vi "Measurement UI.vi"() -> ()   [LabVIEW 2021, in "Single Tone Power Sweep_UI.lvlib"]
uses:
  Single Tone Power Sweep_UI.lvlib
  shared/controls/units - snr.ctl
  shared/controls/units - ratio.ctl
  shared/controls/digital output level units.ctl
  shared/ui/controls/view.ctl
  shared/controls/power measurement method.ctl
  UI State.ctl
  <vilib>/Utility/miscctls.llb/LVBoundsTypeDef.ctl
  <vilib>/Utility/miscctls.llb/LVPoint32TypeDef.ctl
  <vilib>/Utility/miscctls.llb/LVPointTypeDef.ctl
  shared/ui/UI Helpers.lvlib
  shared/audio popup ui/Audio Popup UI.lvlib
  shared/controls/audio controls.lvlib
panel:
  in  "xy graph meas":enum32{"THD+N", "THD", "SNR"}(ring) caption="xy"
  in  "view legend":T1
  out "plot point":string
  out "Sweep graph":cluster{"frequency (Hz)":dbl[], "THD+N":dbl[]}[](graph)
  out "Time domain graph":waveform(dbl)[](graph)
  out "Frequency domain graph":cluster{"f0":dbl, "df":dbl, "data":dbl[]}[](graph)
  out "THD":dbl[](array[numeric])
  out "THD+N":dbl[](array[numeric])
  out "SNR":dbl[](array[numeric])
  out "channel names":string[](array[string])
  in  "digital serial cfg file":string
  in  "power measurement resource":string="PXI1Slot4/ai0"
  out "efficiency (%)":dbl[](array[numeric])
  out "power loss (W)":dbl[](array[numeric])
  out "total output power (W)":dbl[](array[numeric])
  out "input power (W)":dbl[](array[numeric])
  out "power supply current (A)":dbl[](array[numeric])
  out "power supply voltage (V)":dbl[](array[numeric])
  in  "Configuration tab":enum32{"Protocol", "Measurement", "Units"}(tab)
  out "digital serial file name":string
  in  "configure digital serial":bool
  in  "master clock channel list":string caption="Master Clock Channel"
  in  "digital channel list":string caption="Digital Audio Channel"
  in  "output level units 2":T2
  in  "sense resistor (Ohms)":dbl caption="Sense Resistor" format="%#_g Ohms"
  in  "power supply current limit":dbl caption="Current Limit" format="%#_g A"
  in  "power supply voltage":dbl caption="Power Supply Voltage" format="%#_g V"
  in  "power meas resource":refnum<k15> caption="Resource"
  in  "power measurement method":T3 caption="Method"
  in  "output level units":T2
  in  "min settling cycles":u32 caption="Minimum settling cycles"
  in  "min settling time (s)":dbl=0.1 caption="Minimum settling time" format="%#_6ps"
  in  "output sweep number of steps":u32=20000 caption="Number of steps"
  in  "output level start":dbl=20.0 caption="Sweep start" format="%#_6p"
  in  "output level stop":dbl=20000.0 caption="Sweep stop"
  in  "min measurement cycles":u32 caption="Minimum measurement cycles"
  in  "Acquisition channel":tag
  in  "acq sampling rate":dbl=51200.0 caption="Sample rate" format="%#.6pHz"
  in  "min measurement time (s)":dbl=0.1 caption="Minimum measurement time" format="%#_6ps"
  in  "lowpass filter":T4(ring) caption="Lowpass filter"
  in  "highpass filter":enum32{"DC", "AC"}(ring) caption="Highpass filter"
  in  "band start":dbl=20.0 caption="Band start" format="%#_6pHz"
  in  "band stop":dbl=20000.0 caption="Band stop" format="%#_6pHz"
  in  "weighting filter":T5(ring)=enum."A-weighting" caption="Weighting filter"
  in  "load impedance":dbl=4.0 caption="Load impedance" format="%#_6p Ohms"
  in  "output range (pk-pk)":dbl=15.0 caption="Output range" format="%.3p Vpk-pk"
  in  "THD units":T6 caption="THD"
  in  "THD+N units":T6 caption="THD+N"
  in  "SNR units":T7 caption="SNR"
  in  "channel 0 offset":u32=1
  out "fft - data":dbl[](array[numeric])
  out "fft - df":dbl
  out "fft - f0":dbl
  out "wfm - data":dbl[](array[numeric])
  out "wfm - dt":dbl
  out "wfm - t0":dbl
  in  "acq channel":string="PXI1Slot4/ai0"
  in  "signal phase":dbl caption="phase"
  # "hidden controls - used to sync with MeasLink"
  # "hidden indicators"
  # "Digital Serial Settings"
  # "Harware Resource"
  # "Output Sweep"
  # "Filters"
  # "Acquisition"
  # "Power"
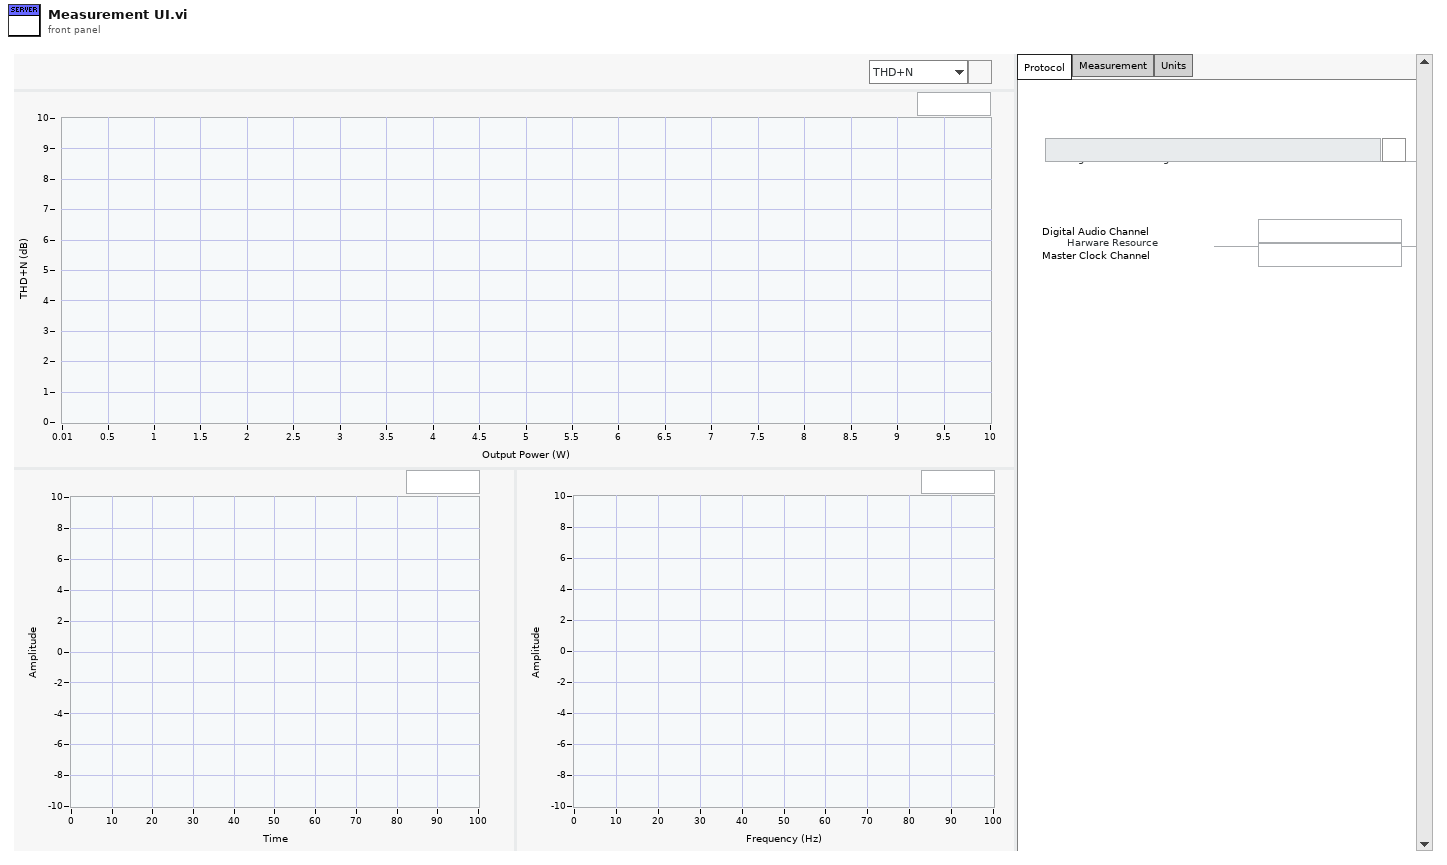
[diagram p1: front panel]
types:
  T1 = typedef "UI Helpers.lvlib/view.ctl" = bool
  T2 = typedef "audio controls.lvlib/digital output level units.ctl" = enum32{"% FS", "dBFS", "V"}
  T3 = typedef "power measurement method.ctl" = enum32{"SMU", "DMM"}
  T4 = enum32{"No filter", "AES17 20kHz", "AES17 40kHz"}
  T5 = enum32{"Linear", "A-weighting", "B-weighting", "C-weighting"}
  T6 = typedef "audio controls.lvlib/units - ratio.ctl" = enum32{"dB", "%", "x/y"}
  T7 = typedef "audio controls.lvlib/units - snr.ctl" = enum32{"dB", "x/y"}
  T8 = typedef "Single Tone Power Sweep_UI.lvlib/UI State.ctl" = cluster{"Graph Size":T9, "Legend Visible":bool, "Mouse Coords":T10, "Visible Plot Id":i32, "PostUI event occurred":bool, "digital serial cfg file":path}
  T9 = typedef "LVBoundsTypeDef.ctl" = cluster{"Width":u32, "Height":u32}
  T10 = typedef "LVPoint32TypeDef.ctl" = cluster{"Horizontal":i32, "Vertical":i32}
  T11 = typedef "LVPointTypeDef.ctl" = cluster{"Horizontal":i16, "Vertical":i16}
  T12 = typedef "Audio Popup UI.lvlib/audio settings.ctl" = cluster{"digital serial file":string}
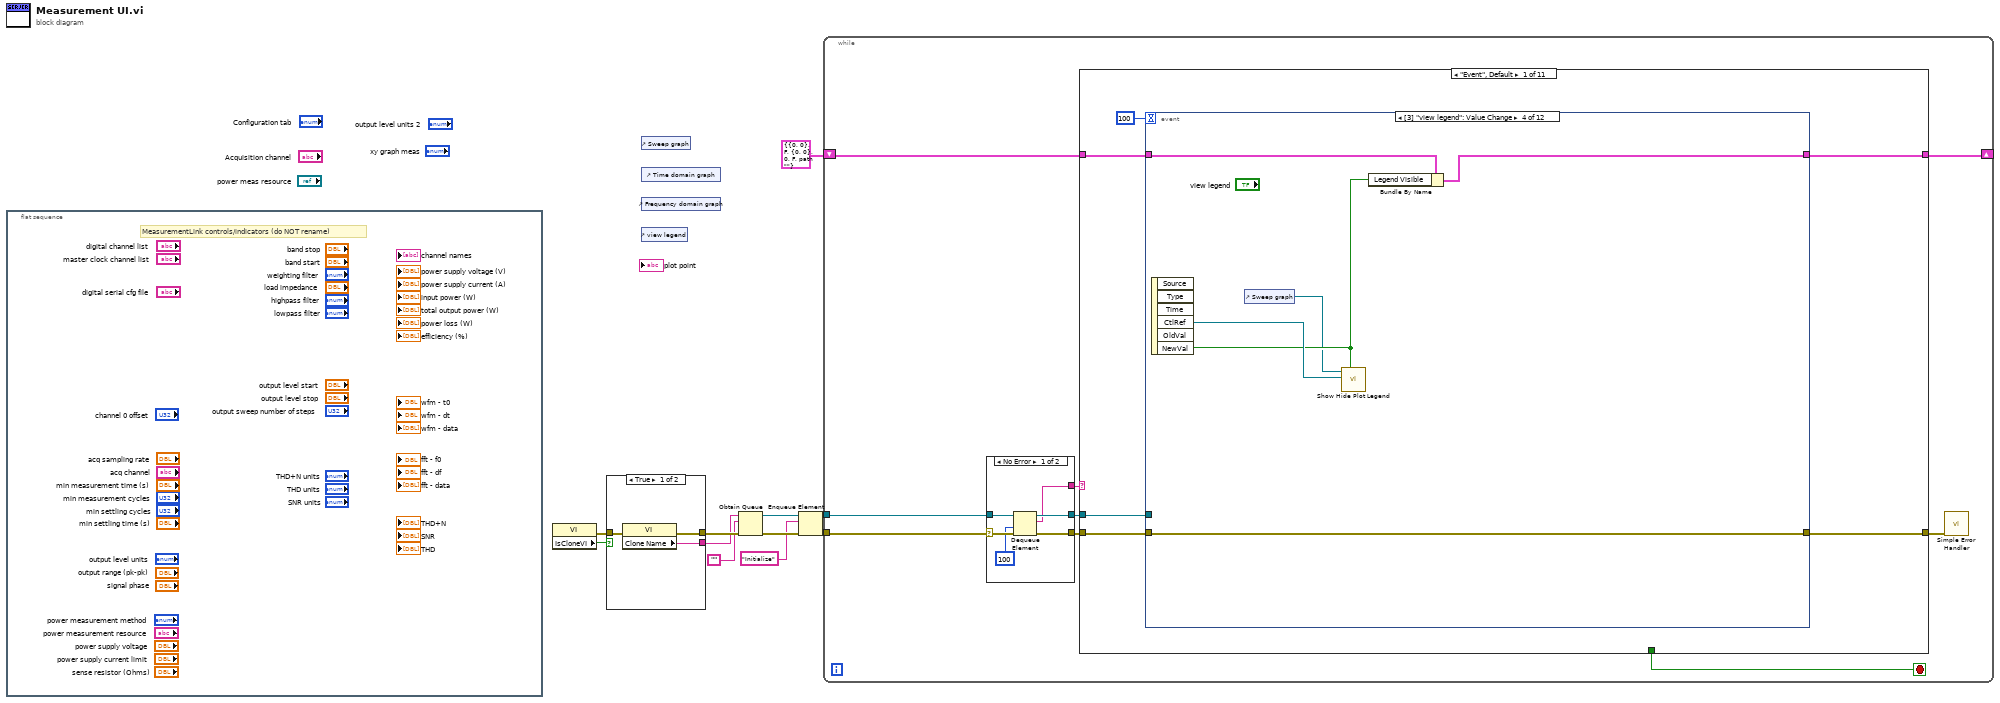
[diagram p0: block diagram]
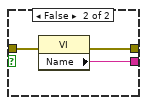
[diagram p2: hidden frame]
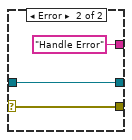
[diagram p3: hidden frame]
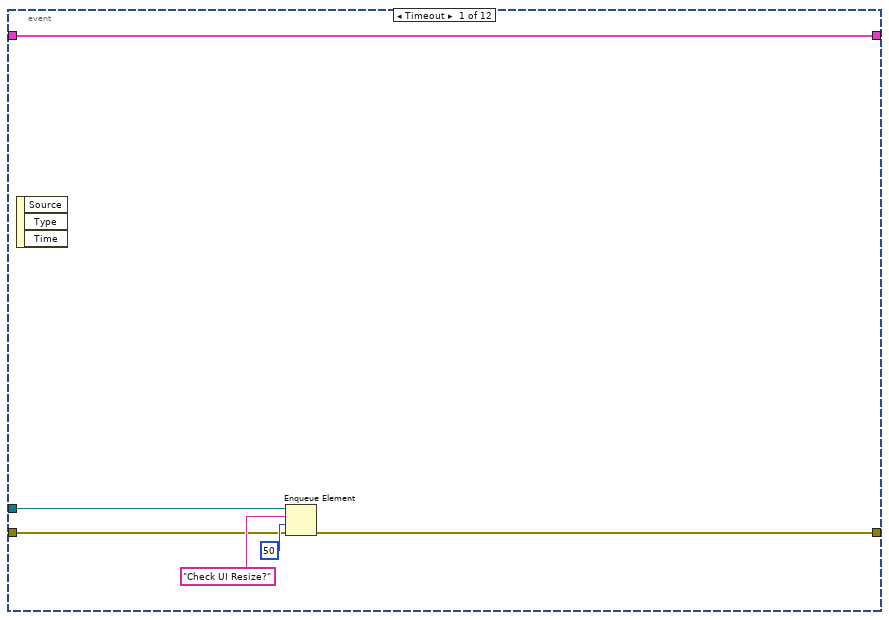
[diagram p4: hidden frame]
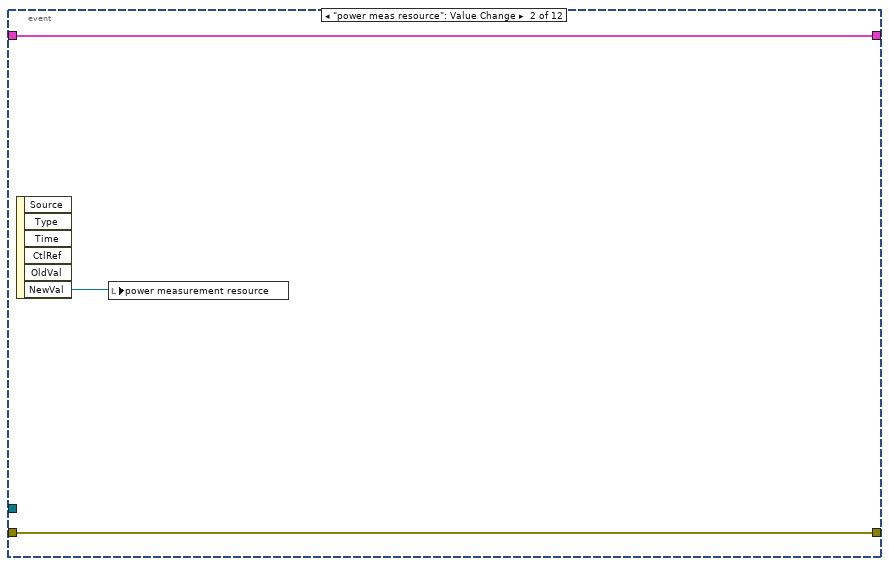
[diagram p5: hidden frame]
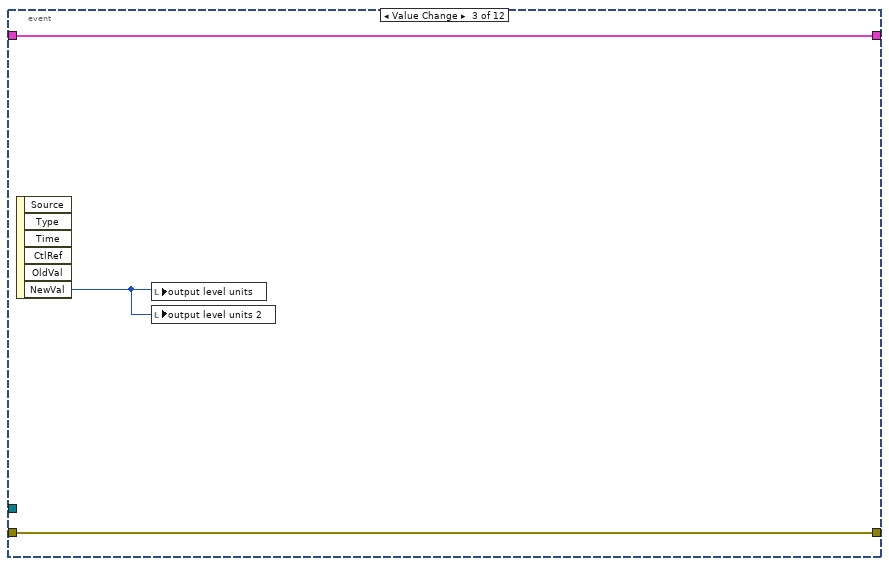
[diagram p6: hidden frame]
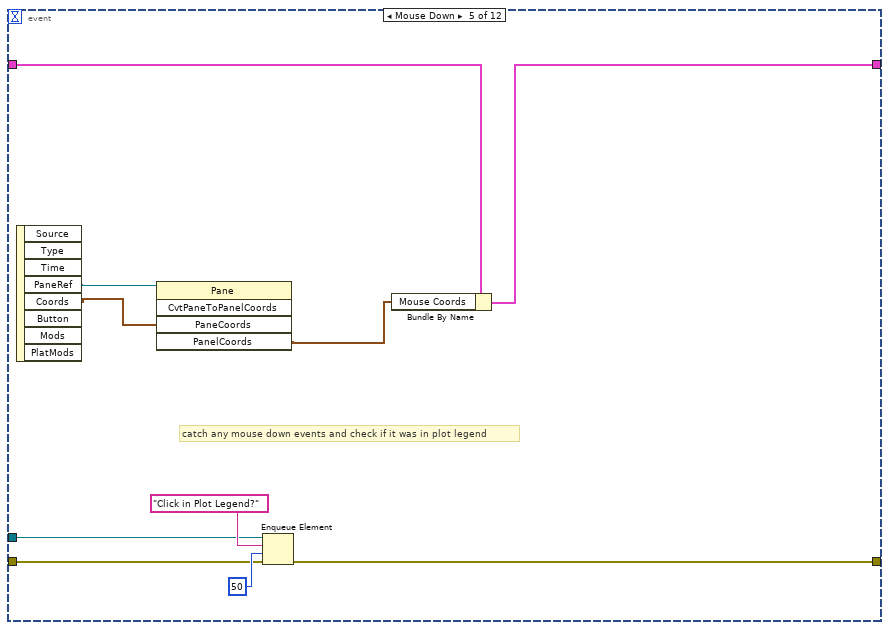
[diagram p7: hidden frame]
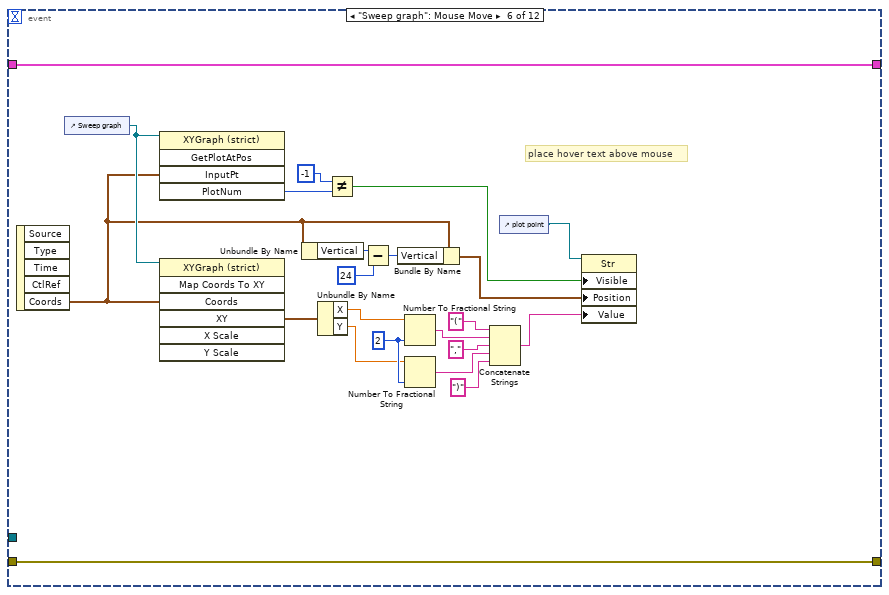
[diagram p8: hidden frame]
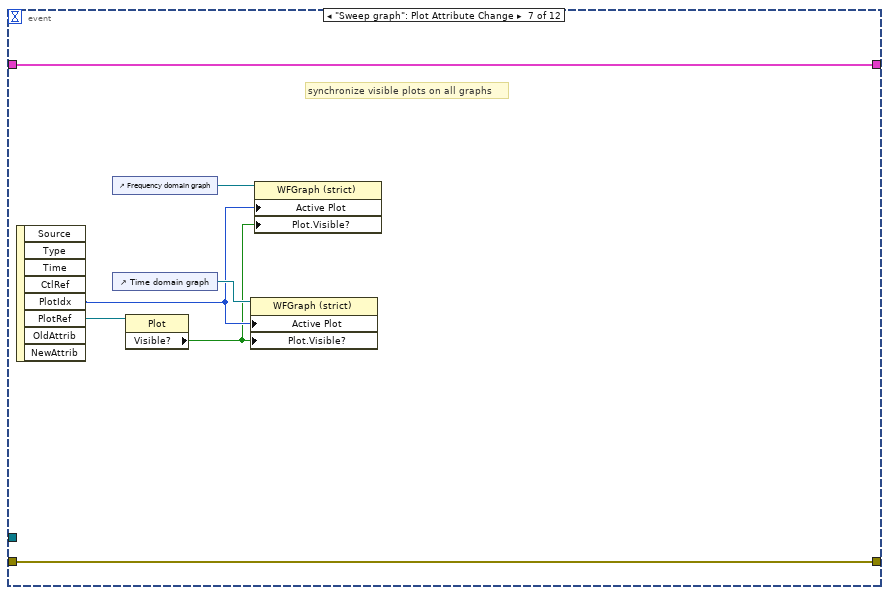
[diagram p9: hidden frame]
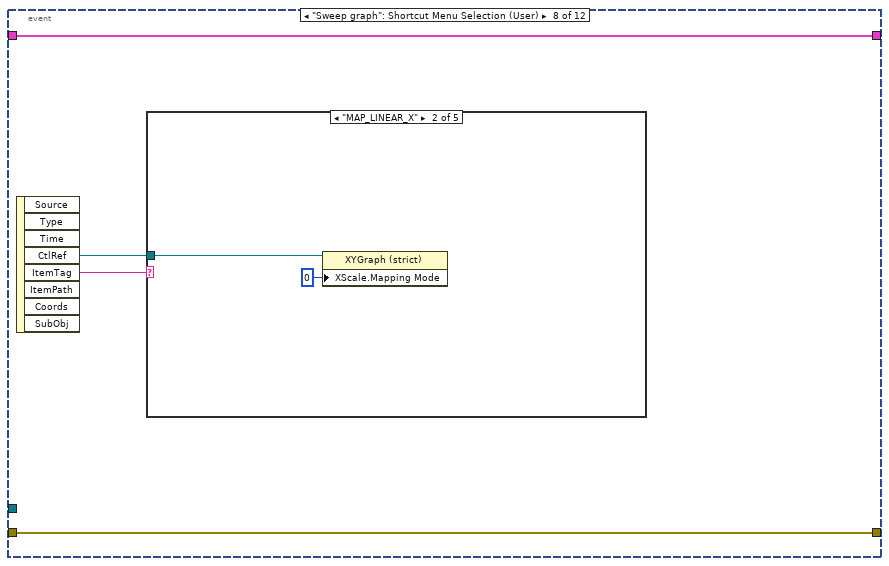
[diagram p10: hidden frame]
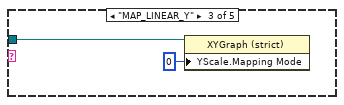
[diagram p12: hidden frame]
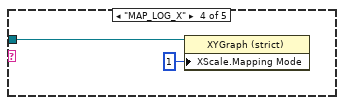
[diagram p13: hidden frame]
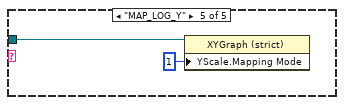
[diagram p14: hidden frame]
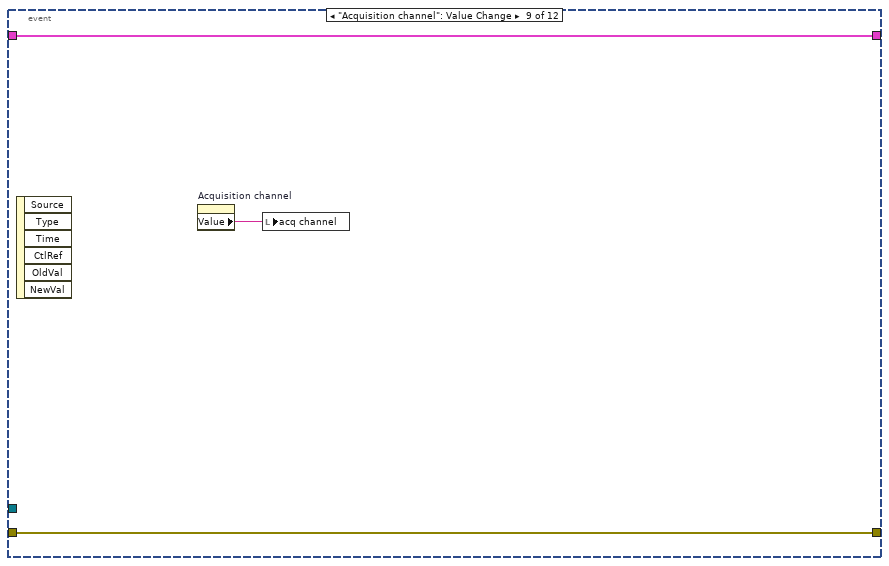
[diagram p15: hidden frame]
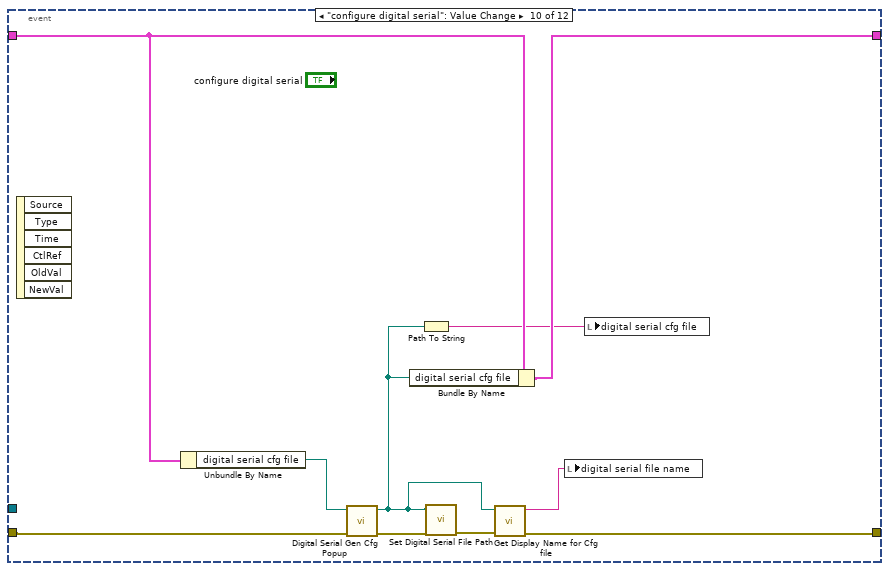
[diagram p16: hidden frame]
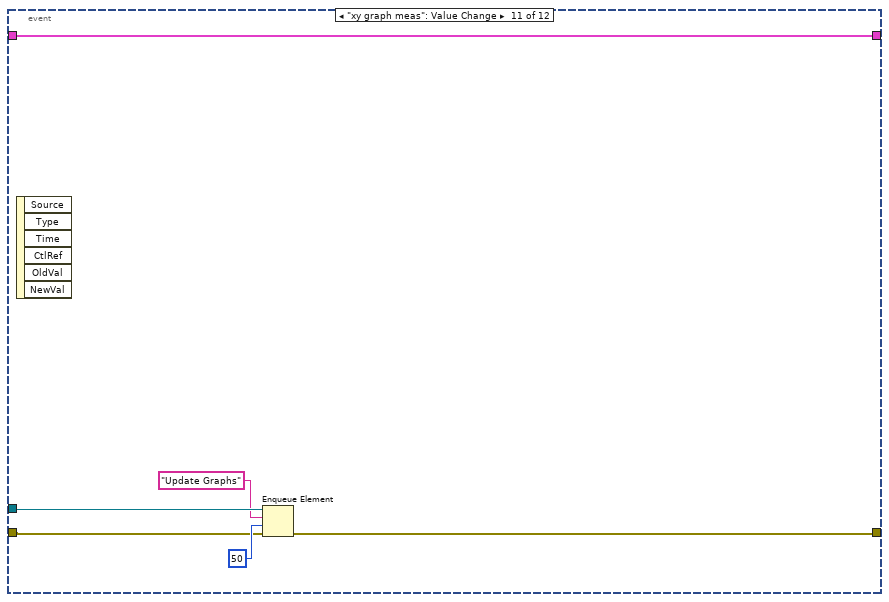
[diagram p17: hidden frame]
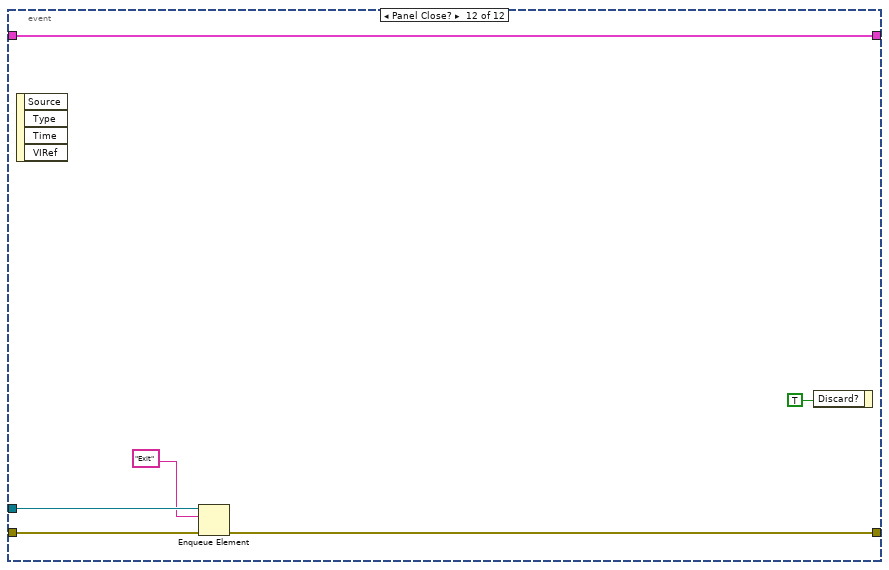
[diagram p18: hidden frame]
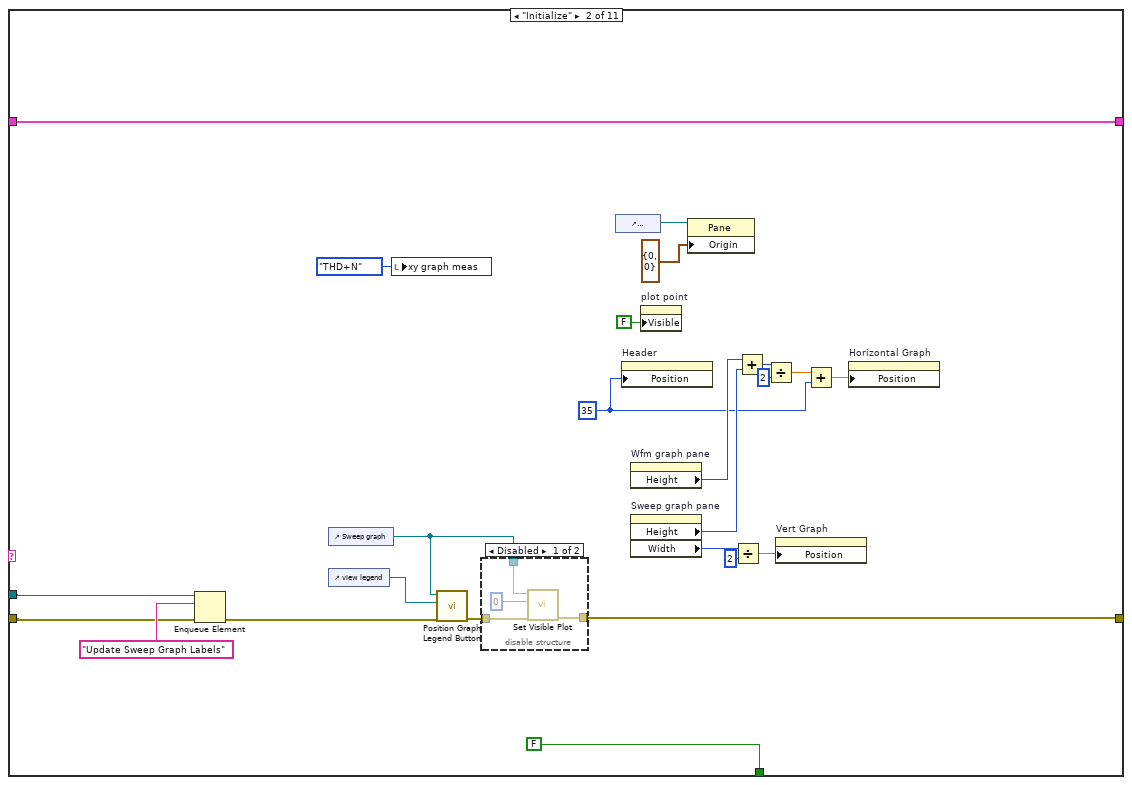
[diagram p19: hidden frame]
diagram:
  n1 = flat-sequence {
    frame #0 {
      # "MeasurementLink controls/indicators (do NOT rename)"
    }
  }
  n2 = property class="VI"() -> (error out=w2:errorcluster, "IsCloneVI"=w3:bool)  [unwired: 2 in, 1 out]
  n3 = case shown="True" w3 {
    tunnel: [w14 w17] -> w11
    tunnel: [w13 w16] -> w10
    tunnel: w2 -> [w12 w15]
    frame True {
      n4 = property class="VI"(error in=w12) -> (error out=w14:errorcluster, "Clone Name"=w13:string)  [unwired: 1 in, 1 out]
    }
    frame False {
      n5 = property class="VI"(error in=w15) -> (error out=w17:errorcluster, "Name"=w16:string)  [unwired: 1 in, 1 out]
    }
  }
  n6 = control-ref of="Sweep graph"() -> ()  [unwired: 1 out]
  n7 = control-ref of="Time domain graph"() -> ()  [unwired: 1 out]
  n8 = control-ref of="Frequency domain graph"() -> ()  [unwired: 1 out]
  n9 = control-ref of="view legend"() -> ()  [unwired: 1 out]
  n10 = Obtain Queue(name (unnamed)=w10, element data type="", error in (no error)=w11) -> (queue out=w7:refnum<queue>, error out=w9:errorcluster)  [unwired: 2 in, 1 out]
  n11 = Enqueue Element(queue=w7, element="Initialize", error in (no error)=w9) -> (queue out=w6:refnum<queue>, error out=w8:errorcluster)  [unwired: 1 in, 1 out]
  n12 = while {
    tunnel: w6 -> [w24]
    shift-right: [w20] -> _
    shift-left: T8 {"Graph Size"={"Width"=0, "Height"=0}, "Legend Visible"=FALSE, "Mouse Coords"={"Horizontal"=0, "Vertical"=0}, "Visible Plot Id"=0, "PostUI event occurred"=FALSE, "digital serial cfg file"=path ""} ("UI State") -> [w19]
    tunnel: w8 -> [w26]
    stop <- w21 stop-if-true
    n13 = case shown="No Error" w26 {
      selector: w26 -> [w32 w35]
      tunnel: [w31 w35] -> w25
      tunnel: w24 -> [w30 w34]
      tunnel: [w29 w34] -> w23
      tunnel: [w28 "Handle Error"] -> w22
      frame No Error {
        n14 = Dequeue Element(queue=w30, timeout in ms (-1)=100, error in (no error)=w32) -> (queue out=w29:refnum<queue>, element=w28:string, error out=w31:errorcluster)  [unwired: 1 out]
      }
      frame Error {
      }
    }
    n15 = case shown="\"Event\", Default" w22 {
      tunnel: w25 -> [w40 w143 w169 w193 w213 w229 w237 w266 w296 w319 w321]
      tunnel: w23 -> [w38 w144 w170 w194 _ _ w236 w267 _ w317 _]
      tunnel: [w41 w147 w168 w192 w212 w220 w231 w265 w296 w314 w321] -> w18
      tunnel: [_ FALSE _ _ _ _ _ _ _ TRUE _] -> w21
      tunnel: [w36 w137 w165 w191 w215 w230 w234 w284 w295 w312 w320] -> w20
      tunnel: w19 -> [w37 w137 w166 w191 w216 w230 w235 w284 w295 w312 w320]
      frame "Event", Default {
        n16 = event shown="[3] \"view legend\": Value Change" {
          selector: _ -> [_ _ _ _ _ _ _ _ _ _ _ _]
          dyn-events: _ -> [_ _ _ _ _ _ _ _ _ _ _ _]
          timeout: 100 -> [_ _ _ _ _ _ _ _ _ _ _ _]
          tunnel: [w44 w50 w53 w59 w65 w91 w97 w102 w111 w114 w124 w133] -> w41
          tunnel: w40 -> [w45 w50 w53 w59 w67 w91 w97 w102 w111 w119 w127 w134]
          tunnel: w38 -> [w43 _ _ _ w66 _ _ _ _ _ w126 w132]
          tunnel: w37 -> [w42 w49 w52 w56 w64 w90 w96 w101 w112 w118 w129 w130]
          tunnel: [w42 w49 w52 w55 w63 w90 w96 w101 w112 w117 w129 w130] -> w36
          event Timeout {
            n17 = event-data() -> ()  [unwired: 1 in, 3 out]
            n18 = Enqueue Element(queue=w43, element="Check UI Resize?", timeout in ms (-1)=50, error in (no error)=w45) -> (error out=w44:errorcluster)  [unwired: 2 out]
          }
          event "power meas resource": Value Change {
            n19 = event-data() -> ("NewVal"=w48:refnum<k15>)  [unwired: 1 in, 5 out]
            n20 = local write "power measurement resource"(w48) -> ()
          }
          event Value Change {
            n21 = event-data() -> ("NewVal"=w51:T2)  [unwired: 1 in, 5 out]
            n22 = local write "output level units"(w51) -> ()
            n23 = local write "output level units 2"(w51) -> ()
          }
          event Value Change {
            n24 = event-data() -> ("CtlRef"=w58:refnum<vi>, "NewVal"=w57:T1)  [unwired: 1 in, 4 out]
            n25 = control-ref of="Sweep graph"() -> (w54:refnum<vi>)
            n26 = call "Show Hide Plot Legend.vi"("show"=w57, "view reference"=w58, "graph reference"=w54) -> ()  [unwired: 8 in, 1 out]
            n27 = Bundle By Name(cluster=w56, "Legend Visible"=w57) -> (w55:T8)
          }
          event Mouse Down {
            # "catch any mouse down events and check if it was in plot legend"
            n28 = event-data() -> ("PaneRef"=w62:refnum<vi>, "Coords"=w61:T10)  [unwired: 1 in, 6 out]
            n29 = invoke class="Pane" method="CvtPaneToPanelCoords"(reference=w62, "PaneCoords"=w61) -> ("PanelCoords"=w60:T11)  [unwired: 3 in, 4 out]
            n30 = Enqueue Element(queue=w66, element="Click in Plot Legend?", timeout in ms (-1)=50, error in (no error)=w67) -> (error out=w65:errorcluster)  [unwired: 2 out]
            n31 = Bundle By Name(cluster=w64, "Mouse Coords"=w60) -> (w63:T8)
          }
          event "Sweep graph": Mouse Move {
            w80 = i16 2 ("precision (6)")
            # "place hover text above mouse"
            n32 = event-data() -> ("Coords"=w70:T10)  [unwired: 1 in, 4 out]
            n33 = control-ref of="Sweep graph"() -> (w71:refnum<vi>)
            n34 = invoke class="XYGraph (strict)" method="GetPlotAtPos"(reference=w71, "InputPt"=w70) -> ("PlotNum"=w88:i32)  [unwired: 3 in, 4 out]
            n35 = invoke class="XYGraph (strict)" method="Map Coords To XY"(reference=w71, "Coords"=w70) -> ("XY"=w89:cluster{"X":dbl, "Y":dbl})  [unwired: 5 in, 6 out]
            n36 = Unbundle By Name(w70) -> ("Vertical"=w75:i32)
            n37 = Unbundle By Name(w89) -> ("X"=w78:dbl, "Y"=w77:dbl)
            n38 = Not Equal?(x=-1, y=w88) -> (x != y?=w86:bool)
            n39 = Subtract(x=w75, y=24) -> (x-y=w74:i32)
            n40 = Bundle By Name(cluster=w70, "Vertical"=w74) -> (w76:T10)
            n41 = Number To Fractional String(number=w78, precision (6)=w80) -> (F-format string=w84:string)  [unwired: 2 in]
            n42 = Number To Fractional String(number=w77, precision (6)=w80) -> (F-format string=w82:string)  [unwired: 2 in]
            n43 = Concatenate Strings("(" ("string"), w84, "," ("string"), w82, ")" ("string")) -> (w79:string)
            n44 = control-ref of="plot point"() -> (w72:refnum<vi>)
            n45 = property on="Property Node" class="Str"(reference=w72, "Visible"=w86, "Position"=w76, "Value"=w79) -> ()  [unwired: 1 in, 2 out]
          }
          event "Sweep graph": Plot Attribute Change {
            # "synchronize visible plots on all graphs"
            n46 = event-data() -> ("PlotIdx"=w93:i32, "PlotRef"=w98:refnum<vi>)  [unwired: 1 in, 6 out]
            n47 = control-ref of="Frequency domain graph"() -> (w94:refnum<vi>)
            n48 = control-ref of="Time domain graph"() -> (w95:refnum<vi>)
            n49 = property class="Plot"(reference=w98) -> ("Visible?"=w92:bool)  [unwired: 1 in, 2 out]
            n50 = property on="Property Node" class="WFGraph (strict)"(reference=w95, "Active Plot"=w93, "Plot.Visible?"=w92) -> ()  [unwired: 1 in, 2 out]
            n51 = property on="Property Node" class="WFGraph (strict)"(reference=w94, "Active Plot"=w93, "Plot.Visible?"=w92) -> ()  [unwired: 1 in, 2 out]
          }
          event "Sweep graph": Shortcut Menu Selection (User) {
            n52 = event-data() -> ("CtlRef"=w99:refnum<vi>, "ItemTag"=w100:string)  [unwired: 1 in, 6 out]
            n53 = case shown="\"MAP_LINEAR_X\"" w100 {
              tunnel: w99 -> [_ w104 w106 w108 w110]
              frame "", Default {
              }
              frame "MAP_LINEAR_X" {
                n54 = property class="XYGraph (strict)"(reference=w104, "XScale.Mapping Mode"=u8 0 ("X Scale.Mapping Mode")) -> ()  [unwired: 1 in, 2 out]
              }
              frame "MAP_LINEAR_Y" {
                n55 = property class="XYGraph (strict)"(reference=w106, "YScale.Mapping Mode"=u8 0 ("X Scale.Mapping Mode")) -> ()  [unwired: 1 in, 2 out]
              }
              frame "MAP_LOG_X" {
                n56 = property class="XYGraph (strict)"(reference=w108, "XScale.Mapping Mode"=u8 1 ("X Scale.Mapping Mode")) -> ()  [unwired: 1 in, 2 out]
              }
              frame "MAP_LOG_Y" {
                n57 = property class="XYGraph (strict)"(reference=w110, "YScale.Mapping Mode"=u8 1 ("X Scale.Mapping Mode")) -> ()  [unwired: 1 in, 2 out]
              }
            }
          }
          event "Acquisition channel": Value Change {
            n58 = event-data() -> ()  [unwired: 1 in, 6 out]
            n59 = property on="Acquisition channel" class="DAQmxName"() -> ("Value"=w113:string)  [unwired: 2 in, 2 out]
            n60 = local write "acq channel"(w113) -> ()
          }
          event "configure digital serial": Value Change {
            n61 = event-data() -> ()  [unwired: 1 in, 6 out]
            n62 = Unbundle By Name(w118) -> ("digital serial cfg file"=w123:path)
            n63 = call "Digital Serial Gen Cfg Popup.vi"("error in (no error)"=w119, "config file in"=w123) -> ("error out"=w122:errorcluster, "config file out"=w120:path)  [unwired: 7 in, 1 out]
            n64 = Bundle By Name(cluster=w118, "digital serial cfg file"=w120) -> (w117:T8)
            n65 = Path To String(path=w120) -> (string=w116:string)
            n66 = call "Set Digital Serial File Path.vi"("error in (no error)"=w122, "digital serial file"=w120) -> ("error out"=w121:errorcluster)  [unwired: 9 in]
            n67 = call "Get Display Name for Cfg file.vi"("error in (no error)"=w121, "file path"=w120) -> ("error out"=w114:errorcluster, "display string"=w115:string)  [unwired: 8 in]
            n68 = local write "digital serial file name"(w115) -> ()
            n69 = local write "digital serial cfg file"(w116) -> ()
          }
          event "xy graph meas": Value Change {
            n70 = event-data() -> ()  [unwired: 1 in, 6 out]
            n71 = Enqueue Element(queue=w126, element="Update Graphs", timeout in ms (-1)=50, error in (no error)=w127) -> (error out=w124:errorcluster)  [unwired: 2 out]
          }
          event Panel Close? {
            n72 = event-data() -> ()  [unwired: 1 in, 4 out]
            n73 = Enqueue Element(queue=w132, element="Exit", error in (no error)=w134) -> (error out=w133:errorcluster)  [unwired: 1 in, 2 out]
            n74 = event-data("Discard?"=TRUE) -> ()  [unwired: 1 in, 1 out]
          }
        }
      }
      frame "Initialize" {
        w141 = 35 ("Splitter Position")
        n75 = Enqueue Element(queue=w144, element="Update Sweep Graph Labels", error in (no error)=w143) -> (error out=w142:errorcluster)  [unwired: 1 in, 2 out]
        n76 = control-ref of="Sweep graph"() -> (w146:refnum<vi>)
        n77 = control-ref of="view legend"() -> (w158:refnum<vi>)
        n78 = local write "xy graph meas"(enum32{"THD+N", "THD", "SNR"}."THD+N" ("xy graph meas")) -> ()
        n79 = call "Position Graph Legend Button.vi"("error in (no error)"=w142, "view legend"=w158, "graph"=w146) -> ("error out"=w148:errorcluster)  [unwired: 8 in]
        n80 = disable-structure shown="Disabled" {
          disable-tunnel: w148 -> [w163 w164]
          disable-tunnel: [w162 w164] -> w147
          disable-tunnel: w146 -> [w161 _]
          frame Disabled {
            n81 = call "Set Visible Plot.vi"("error in (no error)"=w163, "Plot Id"=0, "XYGraph in"=w161) -> ("error out"=w162:errorcluster)  [unwired: 8 in]
          }
          frame Enabled {
          }
        }
        n82 = control-ref of="Configuration Pane"() -> (w140:refnum<vi>)
        n83 = property on="Header" class="Splitter"("Position"=w141) -> ()  [unwired: 2 in, 2 out]
        n84 = property on="Wfm graph pane" class="Pane"() -> ("Height"=w151:u32)  [unwired: 2 in, 2 out]
        n85 = property on="Sweep graph pane" class="Pane"() -> ("Height"=w150:u32, "Width"=w153:u32)  [unwired: 2 in, 2 out]
        n86 = property on="plot point" class="Str"("Visible"=FALSE) -> ()  [unwired: 2 in, 2 out]
        n87 = property class="Pane"(reference=w140, "Origin"=T11 {"Horizontal"=0, "Vertical"=0}) -> ()  [unwired: 1 in, 2 out]
        n88 = Divide(x=w153, y=2) -> (x/y=w152:dbl)
        n89 = Add(x=w151, y=w150) -> (x+y=w149:u32)
        n90 = Divide(x=w149, y=2) -> (x/y=w156:dbl)
        n91 = property on="Vert Graph" class="Splitter"("Position"=w152) -> ()  [unwired: 2 in, 2 out]
        n92 = Add(x=w156, y=w141) -> (x+y=w155:dbl)
        n93 = property on="Horizontal Graph" class="Splitter"("Position"=w155) -> ()  [unwired: 2 in, 2 out]
      }
      frame "Check UI Resize?" {
        n94 = control-ref of="Time domain graph"() -> (w167:refnum<vi>)
        n95 = property on="Property Node" class="WFGraph (strict)"(reference=w167, error in=w169) -> (error out=w175:errorcluster, "Bounds"=w171:T9)  [unwired: 1 out]
        n96 = Unbundle By Name(w166) -> ("Legend Visible"=w173:bool, "Graph Size"=w172:T9)
        n97 = Not Equal?(x=w172, y=w171) -> (x != y?=w174:bool)
        n98 = Bundle By Name(cluster=w166, "Graph Size"=w171) -> (w165:T8)
        n99 = case shown="True" w174 {
          tunnel: w175 -> [w176 w183]
          tunnel: [w176 w178] -> w168
          tunnel: w173 -> [_ w181]
          tunnel: w170 -> [_ w182]
          frame False {
            # "no resize"
          }
          frame True {
            # "panel resized"
            n100 = case shown="True" w181 {
              tunnel: w183 -> [w185 w190]
              tunnel: [w185 w189] -> w180
              tunnel: w182 -> [w184 w188]
              tunnel: [w184 w186] -> w179
              frame False {
              }
              frame True {
                n101 = Enqueue Element(queue=w188, element="Hide Plot Legend", error in (no error)=w190) -> (queue out=w186:refnum<queue>, error out=w189:errorcluster)  [unwired: 1 in, 1 out]
              }
            }
            n102 = Enqueue Element(queue=w179, element="Panel Resize", error in (no error)=w180) -> (error out=w178:errorcluster)  [unwired: 1 in, 2 out]
          }
        }
      }
      frame "Click in Plot Legend?" {
        n103 = Unbundle By Name(w191) -> ("Legend Visible"=w195:bool, "Mouse Coords"=w196:T10)
        n104 = case shown="True" w195 {
          tunnel: w196 -> [_ w203]
          tunnel: w194 -> [_ w200]
          tunnel: w193 -> [w197 w204]
          tunnel: [w197 w199] -> w192
          frame False {
            # "legend not visible; do nothing"
          }
          frame True {
            # "check if mouse down in legend"
            n105 = control-ref of="Sweep graph"() -> (w198:refnum<vi>)
            n106 = call "Check if Click in Graph Legend.vi"("error in (no error)"=w204, "Mouse Coords"=w203, "WaveformGraph"=w198) -> ("error out"=w201:errorcluster, "click in legend?"=w202:bool)  [unwired: 7 in]
            n107 = case shown="True" w202 {
              tunnel: w201 -> [w208 w209]
              tunnel: w200 -> [w207 _]
              tunnel: [w206 w209] -> w199
              frame False {
                n108 = Enqueue Element(queue=w207, element="Hide Plot Legend", error in (no error)=w208) -> (error out=w206:errorcluster)  [unwired: 1 in, 2 out]
              }
              frame True {
                # "inside legend; do nothing"
              }
            }
          }
        }
      }
      frame "Hide Plot Legend" {
        n109 = control-ref of="Sweep graph"() -> (w210:refnum<vi>)
        n110 = control-ref of="view legend"() -> (w211:refnum<vi>)
        n111 = call "Show Hide Plot Legend.vi"("show"=FALSE, "error in (no error)"=w213, "view reference"=w211, "graph reference"=w210) -> ("error out"=w212:errorcluster)  [unwired: 7 in]
        n112 = Bundle By Name(cluster=w216, "Legend Visible"=FALSE ("legend visible")) -> (w215:T8)
      }
      frame "Panel Resize" {
        # "align 'xy meas selection' with 'view legend' boolean"
        n113 = control-ref of="Sweep graph"() -> (w228:refnum<vi>)
        n114 = control-ref of="view legend"() -> (w226:refnum<vi>)
        n115 = call "Position Graph Legend Button.vi"("error in (no error)"=w229, "view legend"=w226, "graph"=w228) -> ("error out"=w227:errorcluster)  [unwired: 8 in]
        n116 = property on="Property Node" class="Bool (strict)"(reference=w226, error in=w227) -> (error out=w224:errorcluster, "Left"=w219:i32)  [unwired: 1 out]
        n117 = control-ref of="xy graph meas"() -> (w225:refnum<vi>)
        n118 = property class="Enum (strict)"(reference=w225, error in=w224) -> (reference out=w223:refnum<vi>, error out=w222:errorcluster, "Width"=w218:u32)
        n119 = Subtract(x=w219, y=w218) -> (x-y=w221:u32)
        n120 = property class="Enum (strict)"(reference=w223, error in=w222, "Left"=w221) -> (error out=w220:errorcluster)  [unwired: 1 out]
      }
      frame "Post UI Update" {
        # "This case will be triggered, after framework updates the User interface with result values."
        n121 = for {
          tunnel: w236 -> [w262]
          shift-right: [w261] -> w232
          shift-left: w237 -> [w263]
          tunnel: string[] ["Update Graphs"] -> [w260] mode=indexing
          n122 = Enqueue Element(queue=w262, element=w260, timeout in ms (-1)=50, error in (no error)=w263) -> (error out=w261:errorcluster)  [unwired: 2 out]
        }
        n123 = Unbundle By Name(w235) -> ("PostUI event occurred"=w233:bool)
        n124 = case shown="False" w233 {
          tunnel: w235 -> [w251 w259]
          tunnel: [w250 w259] -> w234
          tunnel: w232 -> [w245 w258]
          tunnel: [w240 w258] -> w231
          frame False {
            # "Initialize the DAQmx channel control"
            # "do this on first PostUI Event (happens when panel loads)"
            n125 = local read "digital serial cfg file"() -> (w242:string)
            n126 = local read "power measurement resource"() -> (w248:string)
            n127 = Empty String/Path?(string/path=w242) -> (empty?=w241:bool)
            n128 = local read "acq channel"() -> (w247:string)
            n129 = case shown="True" w241 {
              tunnel: w245 -> [w253 w257]
              tunnel: [w253 w255] -> w246
              tunnel: w242 -> [w252 _]
              tunnel: [w252 w254] -> w243
              frame False {
              }
              frame True {
                n130 = call "Get Audio Settings.vi"("error in (no error)"=w257) -> ("error out"=w255:errorcluster, "audio settings"=w256:T12)  [unwired: 9 in]
                n131 = Unbundle By Name(w256) -> ("digital serial file"=w254:string)
              }
            }
            n132 = local write "power meas resource"(w248) -> ()
            n133 = property on="Acquisition channel" class="DAQmxName"("Value"=w247) -> ()  [unwired: 2 in, 2 out]
            n134 = String To Path(string=w243) -> (path=w244:path)
            n135 = local write "digital serial cfg file"(w243) -> ()
            n136 = call "Get Display Name for Cfg file.vi"("error in (no error)"=w246, "file path"=w244) -> ("error out"=w240:errorcluster, "display string"=→"digital serial file name":string)  [unwired: 8 in]
            n137 = Bundle By Name(cluster=w251, "PostUI event occurred"=TRUE, "digital serial cfg file"=w244) -> (w250:T8)
          }
          frame True {
          }
        }
      }
      frame "Update Graphs" {
        n138 = local read "channel names"() -> (w274:string[])
        n139 = disable-structure shown="Disabled" {
          frame Disabled {
            # "maybe use for debugging ???"
            n140 = local read "power supply voltage (V)"() -> ()  [unwired: 1 out]
            n141 = local read "power supply current (A)"() -> ()  [unwired: 1 out]
          }
          frame Enabled {
          }
        }
        n142 = control-ref of="Sweep graph"() -> (w283:refnum<vi>)
        n143 = Array Size(array=w274) -> (size(s)=w282:i32)
        n144 = Enqueue Element(queue=w267, element="Update Sweep Graph Labels", error in (no error)=w266) -> (error out=w265:errorcluster)  [unwired: 1 in, 2 out]
        n145 = property class="XYGraph (strict)"(reference=w283, "LegNumRows"=w282, "LegScrollVis"=FALSE ("Legend:Scrollbar Visible")) -> ()  [unwired: 1 in, 2 out]
        n146 = for {
          tunnel: w274 -> [w291] mode=indexing
          tunnel: w283 -> [w290]
          i -> [w292]
          n147 = property on="Property Node" class="XYGraph (strict)"(reference=w290, "Active Plot"=w292, "Plot.Plot Name"=w291, "Plot.Point Style"=u8 5, "Plot.Visible?"=TRUE ("Plot.Visible")) -> ()  [unwired: 1 in, 2 out]
        }
        n148 = local read "xy graph meas"() -> (w269:enum32{"THD+N", "THD", "SNR"})
        n149 = local read "fft - data"() -> (w271:dbl[])
        n150 = local read "wfm - data"() -> (w277:dbl[])
        n151 = local read "fft - df"() -> (w273:dbl)
        n152 = local read "fft - f0"() -> (w272:dbl)
        n153 = local read "wfm - dt"() -> (w276:dbl)
        n154 = local read "total output power (W)"() -> (w279:dbl[])
        n155 = case shown="\"SNR\"" w269 {
          tunnel: [w285 w286 w287] -> w278
          frame "THD+N", Default {
            n156 = local read "THD+N"() -> (w285:dbl[])
          }
          frame "THD" {
            n157 = local read "THD"() -> (w286:dbl[])
          }
          frame "SNR" {
            n158 = local read "SNR"() -> (w287:dbl[])
          }
        }
        n159 = call "Array to Wfm (N Ch).vi"("channel names"=w274, "dt"=w276, "array"=w277) -> ("waveforms"=→"Time domain graph":waveform(dbl)[])  [unwired: 8 in]
        n160 = call "Array to Spectra (N Ch).vi"("channel names"=w274, "df"=w273, "f0"=w272, "data"=w271) -> ("spectra"=→"Frequency domain graph":cluster{"f0":dbl, "df":dbl, "data":dbl[]}[])  [unwired: 7 in]
        n161 = call "Array to XY (N Ch).vi"("channel names"=w274, "Y data"=w278, "X data"=w279) -> ("XY plots"=→"Sweep graph":cluster{"X data":dbl[], "Y data":dbl[]}[])  [unwired: 8 in]
      }
      frame "Update Sweep Graph Labels" {
        n162 = local read "xy graph meas"() -> (w294:enum32{"THD+N", "THD", "SNR"})
        n163 = case shown="\"SNR\"" w294 {
          tunnel: [w297 w302 w307] -> w293
          frame "THD+N", Default {
            n164 = local read "THD+N units"() -> (w300:T6)
            n165 = Format Into String(w300) -> (resulting string=w299:string)  [unwired: 3 in, 1 out]
            n166 = Concatenate Strings("THD+N (", w299, ")" ("string")) -> (w297:string)
          }
          frame "THD" {
            n167 = local read "THD units"() -> (w305:T6)
            n168 = Format Into String(w305) -> (resulting string=w304:string)  [unwired: 3 in, 1 out]
            n169 = Concatenate Strings("THD (", w304, ")" ("string")) -> (w302:string)
          }
          frame "SNR" {
            n170 = local read "SNR units"() -> (w310:T7)
            n171 = Format Into String(w310) -> (resulting string=w309:string)  [unwired: 3 in, 1 out]
            n172 = Concatenate Strings("SNR (", w309, ")" ("string")) -> (w307:string)
          }
        }
        n173 = property on="Sweep graph" class="XYGraph (strict)"("YScale.NameLbl.Text"=w293) -> ()  [unwired: 2 in, 2 out]
      }
      frame "Exit" {
        # "This case is triggered to close the User Interface from framework"
        n174 = Flush Queue(queue=w317, error in (no error)=w319) -> (queue out=w316:refnum<queue>, error out=w315:errorcluster)  [unwired: 1 out]
        n175 = Release Queue(queue=w316, force destroy? (F)=TRUE, error in (no error)=w315) -> (error out=w314:errorcluster)  [unwired: 2 out]
      }
      frame "Handle Error" {
      }
    }
    n176 = call <vilib>:"Simple Error Handler.vi"("error in (no error)"=w18) -> ()  [unwired: 4 in, 5 out]
  }
